vi "Setup.Hide.vi"(8 "error in (no error)":errorcluster, 10 "Name":refnum<vi>, 11 "Value":refnum<vi>) -> (0 "error out":errorcluster)   [LabVIEW 2015, in "Workspace.Obejct.Radio.lvlib"]
uses:
  Workspace.Obejct.Radio.lvlib
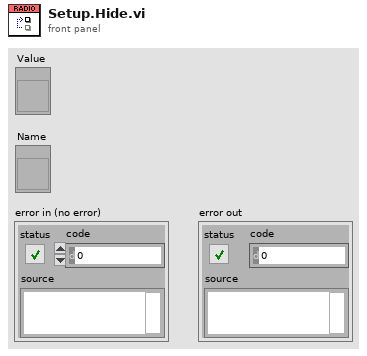
[diagram p1: front panel]
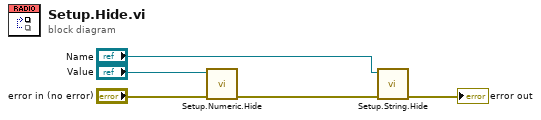
[diagram p0: block diagram]
diagram:
  n1 = call "Setup.Numeric.Hide.vi"("error in (no error)"="error in (no error)", "Digital in"="Value") -> ("error out"=w3:errorcluster)  [unwired: 9 in]
  n2 = call "Setup.String.Hide.vi"("error in (no error)"=w3, "String in"="Name") -> ("error out"=→"error out":errorcluster)  [unwired: 9 in]
